vi "calculate AO2 zy waveform.vi"(8 "error in (no error)":errorcluster, 11 "NI in":refnum<class "NI.lvclass">) -> (0 "error out":errorcluster, 3 "NI out":refnum<class "NI.lvclass">)   [LabVIEW 2021, in "NI.lvlib" / "NI.lvclass"]
uses:
  NI.lvclass
  NI.lvclass/NI.ctl
  <vilib>/Analysis/NI_AALPro.lvlib
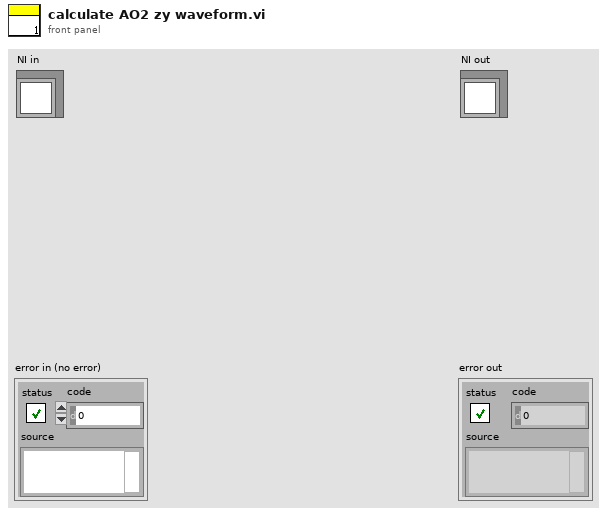
[diagram p1: front panel]
types:
  T1 = typedef "NI.lvlib/NI.lvclass/NI task parameters.ctl" = cluster{"exposure time":dbl, "camera H":dbl, "y line #":dbl, "flyback line #":dbl, "y pixel size":dbl, "z scan #":dbl, "z step size":dbl, "z offset":dbl, "laser all on?":bool, "laser option":bool[]}
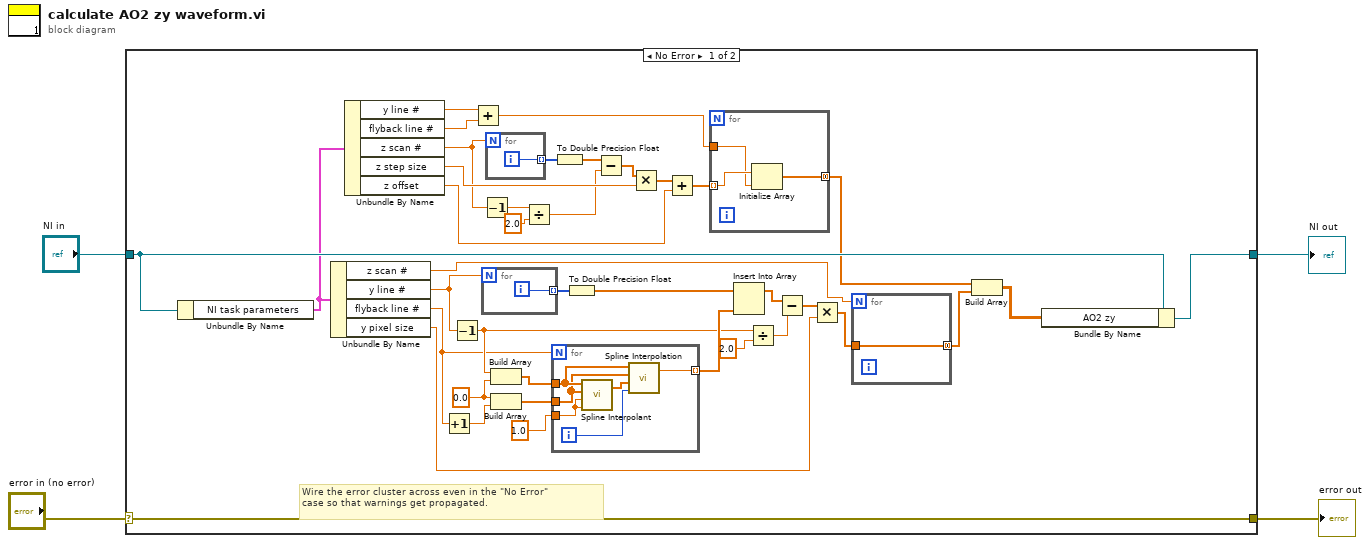
[diagram p0: block diagram]
diagram:
  n1 = case shown="No Error" "error in (no error)" {
    selector: "error in (no error)" -> [w43 w57]
    tunnel: [w43 w57] -> w2
    tunnel: [w25 w56] -> w1
    tunnel: "NI in" -> [w26 w56]
    frame No Error {
      w38 = 0.0 ("element")
      # "Wire the error cluster across even in the \"No Error\"\ncase so that warnings get propagated."
      n2 = Unbundle By Name(w26) -> ("NI task parameters"=w13:T1)
      n3 = Unbundle By Name(w13) -> ("z scan #"=w6:dbl, "y line #"=w30:dbl, "flyback line #"=w29:dbl, "y pixel size"=w27:dbl)
      n4 = Unbundle By Name(w13) -> ("y line #"=w12:dbl, "flyback line #"=w11:dbl, "z scan #"=w15:dbl, "z step size"=w21:dbl, "z offset"=w23:dbl)
      n5 = Increment(x=w29) -> (x+1=w40:dbl)
      n6 = Decrement(x=w30) -> (x-1=w32:dbl)
      n7 = Add(x=w12, y=w11) -> (x+y=w9:dbl)
      n8 = Decrement(x=w15) -> (x-1=w16:dbl)
      n9 = for {
        N: w30 -> [_]
        tunnel: [w55] -> w42 mode=indexing
        i -> [w55]
      }
      n10 = for {
        N: w15 -> [_]
        tunnel: [w48] -> w14 mode=indexing
        i -> [w48]
      }
      n11 = Build Array(w32, w38) -> (w41:dbl[])
      n12 = Build Array(w38, w40) -> (w39:dbl[])
      n13 = Divide(x=w16, y=2.0) -> (x/y=w19:dbl)
      n14 = for {
        N: w29 -> [_]
        tunnel: w41 -> [w52]
        tunnel: w39 -> [w51]
        tunnel: 1.0 ("final boundary") -> [w53]
        tunnel: [w49] -> w35 mode=indexing
        i -> [w50]
        n15 = call <vilib>:"Spline Interpolant.vi"("final boundary"=w53, "initial boundary"=w53, "X"=w51, "Y"=w52) -> ("Interpolant"=w54:dbl[])  [unwired: 1 out]
        n16 = call <vilib>:"Spline Interpolation.vi"("x value"=w50, "Interpolant"=w54, "X"=w51, "Y"=w52) -> ("interpolation value"=w49:dbl)  [unwired: 1 out]
      }
      n17 = To Double Precision Float(number=w14) -> (double precision float=w18:dbl[])
      n18 = To Double Precision Float(number=w42) -> (double precision float=w36:dbl[])
      n19 = Subtract(x=w18, y=w19) -> (x-y=w20:dbl[])
      n20 = Multiply(x=w20, y=w21) -> (x*y=w22:dbl[])
      n21 = Add(x=w22, y=w23) -> (x+y=w10:dbl[])
      n22 = for {
        tunnel: w10 -> [w47] mode=indexing
        tunnel: w9 -> [w46]
        tunnel: [w45] -> w8 mode=concatenating
        n23 = Initialize Array(w47, w46) -> (w45:dbl[])
      }
      n24 = Insert Into Array(array=w36, new element=w35) -> (w34:dbl[])  [unwired: 1 in]
      n25 = Divide(x=w32, y=2.0) -> (x/y=w31:dbl)
      n26 = Subtract(x=w34, y=w31) -> (x-y=w28:dbl[])
      n27 = Multiply(x=w28, y=w27) -> (x*y=w7:dbl[])
      n28 = for {
        N: w6 -> [_]
        tunnel: w7 -> [w44]
        tunnel: [w44] -> w5 mode=concatenating
      }
      n29 = Build Array(w8, w5) -> (w24:dbl[][])
      n30 = Bundle By Name(cluster=w26, "AO2 zy"=w24) -> (w25:refnum<class "NI.lvclass">)
    }
    frame Error {
    }
  }
  "error out" <- w2
  "NI out" <- w1
